vi "Results_filename_checker.vi"(4 "Filelength":i32=25, 5 "Warn if Already Exists":bool, 6 "Comment":string, 7 "Show Error handler":bool=TRUE, 8 "Results file":path) -> (0 "exists?":bool, 1 "Error String":string, 2 "cancelled":bool, 3 "Results file output":path)   [LabVIEW 2014]
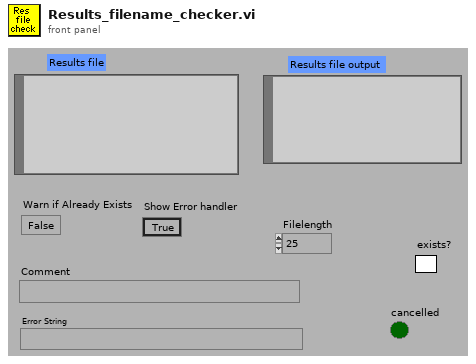
[diagram p1: front panel]
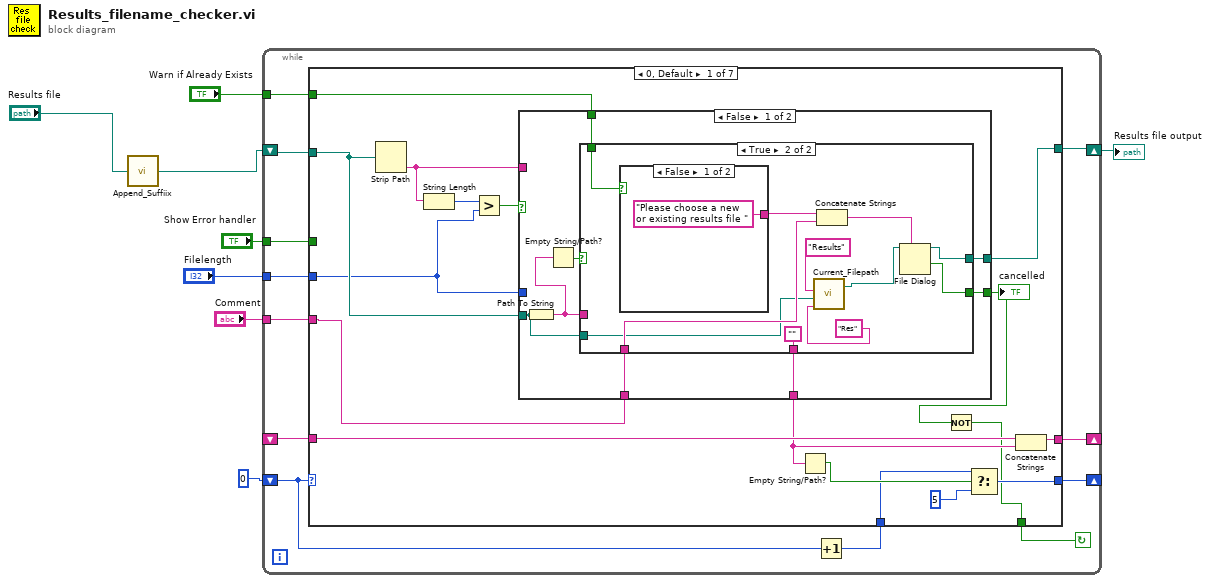
[diagram p0: block diagram]
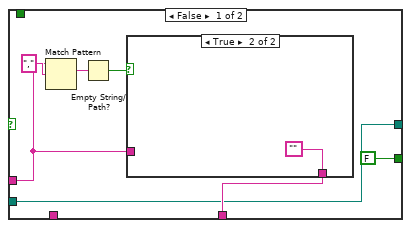
[diagram p2: hidden frame]
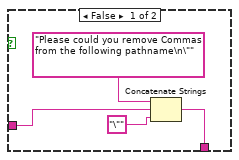
[diagram p3: hidden frame]
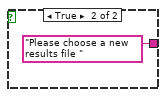
[diagram p4: hidden frame]
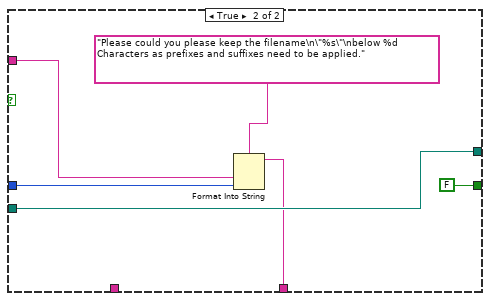
[diagram p5: hidden frame]
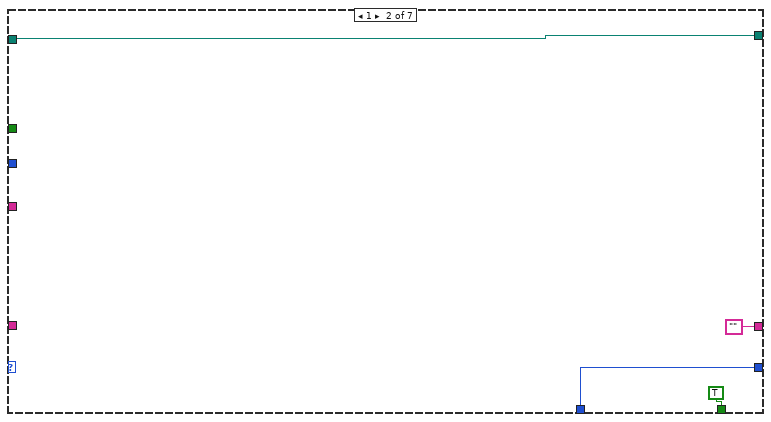
[diagram p6: hidden frame]
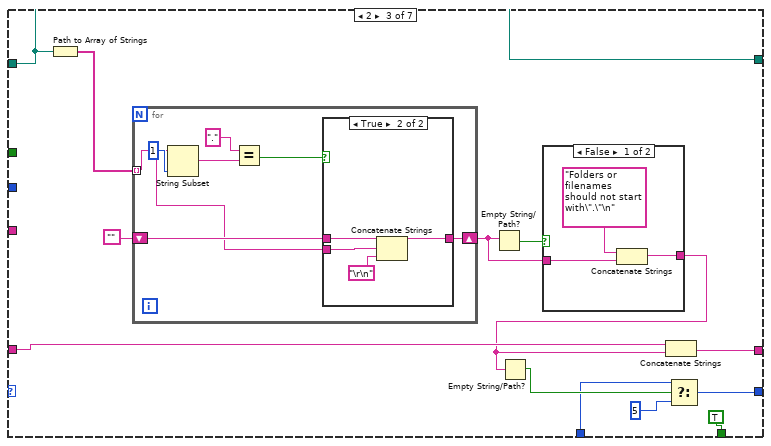
[diagram p7: hidden frame]
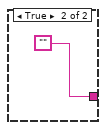
[diagram p8: hidden frame]
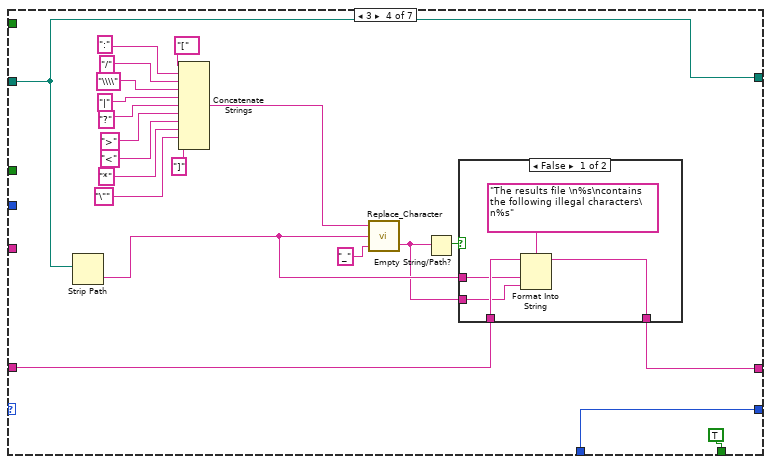
[diagram p10: hidden frame]
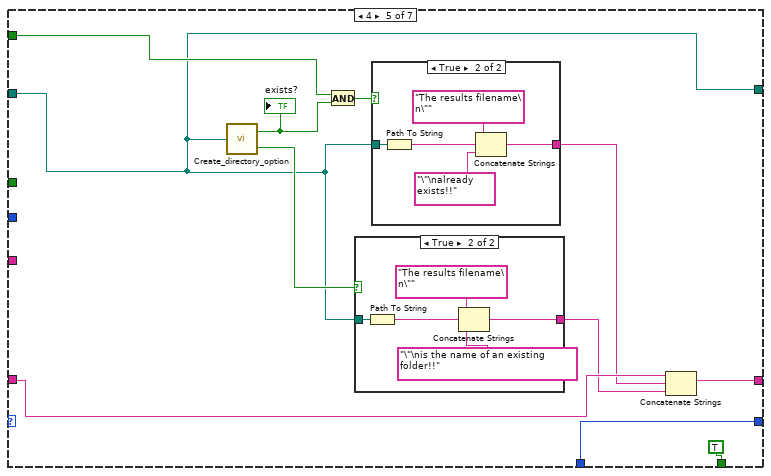
[diagram p12: hidden frame]
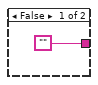
[diagram p13: hidden frame]
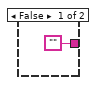
[diagram p14: hidden frame]
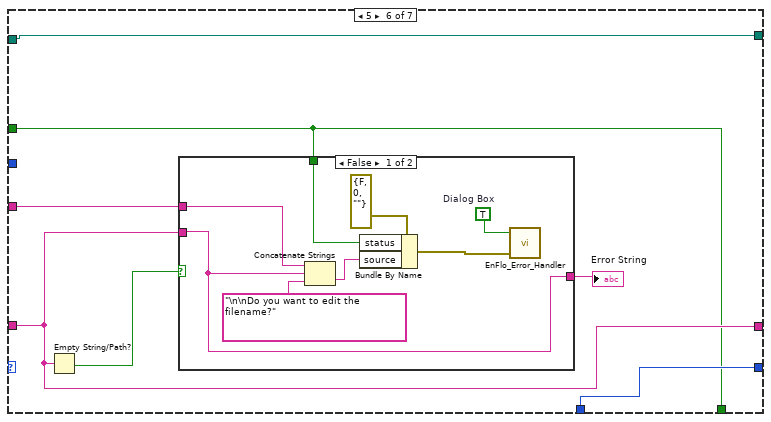
[diagram p15: hidden frame]
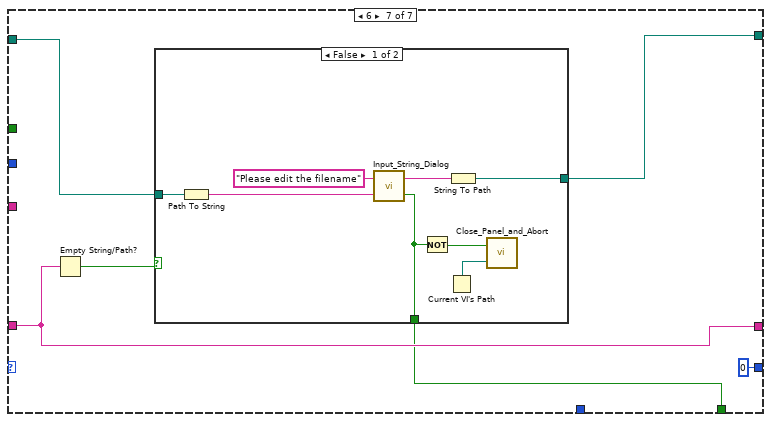
[diagram p17: hidden frame]
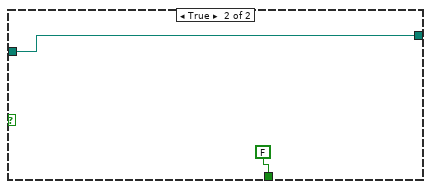
[diagram p18: hidden frame]
diagram:
  n1 = call "Append_Suffiix.vi"("Results file"="Results file") -> ("appended path"=w1:path)
  n2 = while {
    shift-left: 0 -> [w16]
    shift-right: [w12] -> _
    shift-left: _ -> [w15]
    shift-right: [w14] -> _
    tunnel: "Show Error handler" -> [w17]
    shift-left: w1 -> [w20]
    shift-right: [w19] -> w8
    tunnel: "Warn if Already Exists" -> [w11]
    tunnel: "Comment" -> [w10]
    tunnel: "Filelength" -> [w9]
    stop <- w18 continue-if-true
    n3 = Increment(x=w16) -> (x+1=w13:i32)
    n4 = case shown="0, Default" w16 {
      tunnel: w20 -> [w26 w77 w81 w117 w137 w161 w180]
      tunnel: [w27 w77 w81 w117 w137 w161 w181] -> w19
      tunnel: [w23 TRUE ("Ok Out") TRUE ("Ok Out") TRUE ("Ok Out") TRUE ("Ok Out") w162 w178] -> w18
      tunnel: w17 -> [_ _ _ _ _ w162 _]
      tunnel: w15 -> [w36 _ w86 w115 w144 w164 w179]
      tunnel: [w35 "" w84 w114 w143 w164 w179] -> w14
      tunnel: w13 -> [w32 w79 w83 w113 w141 w163 _]
      tunnel: [w30 w79 w82 w113 w141 w163 0 ("f")] -> w12
      tunnel: w11 -> [w25 _ _ _ w138 _ _]
      tunnel: w10 -> [w22 _ _ _ _ w160 _]
      tunnel: w9 -> [w21 _ _ _ _ _ _]
      frame 0, Default {
        n5 = Strip Path(path=w26) -> (name=w29:string)  [unwired: 1 out]
        n6 = String Length(string=w29) -> (length=w28:i32)
        n7 = Greater?(x=w28, y=w21) -> (0:w37:bool)
        n8 = case shown="False" w37 {
          tunnel: w26 -> [w41 w76]
          tunnel: w29 -> [_ w74]
          tunnel: [w45 w72] -> w34
          tunnel: [w42 w76] -> w27
          tunnel: w25 -> [w40 _]
          tunnel: [w39 FALSE ("cancelled")] -> w24
          tunnel: w22 -> [w38 _]
          tunnel: w21 -> [_ w73]
          frame False {
            n9 = Path To String(path=w41) -> (string=w44:string)
            n10 = Empty String/Path?(string/path=w44) -> (empty?=w43:bool)
            n11 = case shown="True" w43 {
              tunnel: [w52 ""] -> w45
              tunnel: w44 -> [w48 _]
              tunnel: [w47 w63] -> w42
              tunnel: w41 -> [w47 w60]
              tunnel: w40 -> [_ w67]
              tunnel: [FALSE ("cancelled") w62] -> w39
              tunnel: w38 -> [_ w65]
              frame False {
                n12 = Match Pattern(string=w48, regular expression=",") -> (match substring=w50:string)  [unwired: 4 out]
                n13 = Empty String/Path?(string/path=w50) -> (empty?=w49:bool)
                n14 = case shown="True" w49 {
                  tunnel: w48 -> [w55 _]
                  tunnel: [w54 ""] -> w52
                  frame False {
                    n15 = Concatenate Strings("Please could you remove Commas from the following pathname\n\"", w55, "\"") -> (w54:string)
                  }
                  frame True {
                  }
                }
              }
              frame True {
                n16 = case shown="False" w67 {
                  tunnel: ["Please choose a new or existing results file " ("prompt") "Please choose a new results file " ("prompt")] -> w66
                  frame False {
                  }
                  frame True {
                  }
                }
                n17 = call "Current_Filepath.vi"("Short_Name"="Res" ("Data Type"), "Filename in"=w60, "Data Type"="Results") -> ("Directory"=w59:path)  [unwired: 1 in, 1 out]
                n18 = Concatenate Strings(w66, w65) -> (w64:string)
                n19 = File Dialog(7:w64, 11:w59) -> (1:w62:bool, 3:w63:path)  [unwired: 5 in, 2 out]
              }
            }
          }
          frame True {
            n20 = Format Into String(format string="Please could you please keep the filename\n\"%s\"\nbelow %d Characters as prefixes and suffixes need to be applied.", w74, w73) -> (resulting string=w72:string)  [unwired: 2 in, 1 out]
          }
        }
        "cancelled" <- w24
        n21 = Empty String/Path?(string/path=w34) -> (empty?=w33:bool)
        n22 = Not(x=w24) -> (.not. x?=w23:bool)
        n23 = Select(t=w32, s=w33, f=5) -> (s? t:f=w30:i32)
        n24 = Concatenate Strings(w36, w34) -> (w35:string)
      }
      frame 1 {
      }
      frame 2 {
        n25 = Path to Array of Strings(0:w81) -> (2:w91:string[])  [unwired: 1 out]
        n26 = for {
          tunnel: w91 -> [w99] mode=indexing
          shift-right: [w98] -> w89
          shift-left: "" -> [w100]
          n27 = String Subset(string=w99, length (rest)=1 ("length")) -> (substring=w103:string)  [unwired: 1 out]
          n28 = Equal?(x=".", y=w103) -> (x = y?=w101:bool)
          n29 = case shown="True" w101 {
            tunnel: w100 -> [w105 w109]
            tunnel: w99 -> [_ w108]
            tunnel: [w105 w107] -> w98
            frame False {
            }
            frame True {
              n30 = Concatenate Strings(w109, w108, "\r\n") -> (w107:string)
            }
          }
        }
        n31 = Empty String/Path?(string/path=w89) -> (empty?=w90:bool)
        n32 = case shown="False" w90 {
          tunnel: [w94 ""] -> w85
          tunnel: w89 -> [w95 _]
          frame False {
            n33 = Concatenate Strings("Folders or filenames should not start with\".\"\n", w95) -> (w94:string)
          }
          frame True {
          }
        }
        n34 = Empty String/Path?(string/path=w85) -> (empty?=w88:bool)
        n35 = Concatenate Strings(w86, w85) -> (w84:string)
        n36 = Select(t=w83, s=w88, f=5) -> (s? t:f=w82:i32)
      }
      frame 3 {
        n37 = Strip Path(path=w117) -> (name=w111:string)  [unwired: 1 out]
        n38 = Concatenate Strings("[" ("Substring"), ":", "/", "\\\\", "|", "?", ">", "<", "*", "\"", "]" ("Substring")) -> (w119:string)
        n39 = call "Replace_Character.vi"("Replace with"="_", "Input String"=w111, "Search For"=w119) -> ("Matched Characters"=w110:string)  [unwired: 1 out]
        n40 = Empty String/Path?(string/path=w110) -> (empty?=w116:bool)
        n41 = case shown="False" w116 {
          tunnel: w115 -> [w134 w136]
          tunnel: [w133 w136] -> w114
          tunnel: w111 -> [w132 _]
          tunnel: w110 -> [w131 _]
          frame False {
            n42 = Format Into String(format string="The results file \n%s\ncontains the following illegal characters\n%s" ("Format String"), initial string=w134, w132, w131) -> (resulting string=w133:string)  [unwired: 1 in, 1 out]
          }
          frame True {
          }
        }
      }
      frame 4 {
        n43 = call "Create_directory_option.vi"("Filename"=w137) -> ("Path is to existing File"=w146:bool, "Path is to existing Directory"=w139:bool)
        "exists?" <- w146
        n44 = And(x=w138, y=w146) -> (x .and. y?=w145:bool)
        n45 = case shown="True" w139 {
          tunnel: w137 -> [_ w151]
          tunnel: ["" w150] -> w140
          frame False {
          }
          frame True {
            n46 = Path To String(path=w151) -> (string=w149:string)
            n47 = Concatenate Strings("The results filename\n\"", w149, "\"\nis the name of an existing folder!!") -> (w150:string)
          }
        }
        n48 = case shown="True" w145 {
          tunnel: w137 -> [_ w157]
          tunnel: ["" w156] -> w142
          frame False {
          }
          frame True {
            n49 = Path To String(path=w157) -> (string=w155:string)
            n50 = Concatenate Strings("The results filename\n\"", w155, "\"\nalready exists!!") -> (w156:string)
          }
        }
        n51 = Concatenate Strings(w144, w142, w140) -> (w143:string)
      }
      frame 5 {
        n52 = Empty String/Path?(string/path=w164) -> (empty?=w166:bool)
        n53 = case shown="False" w166 {
          tunnel: w164 -> [w168 w175]
          tunnel: [w168 w175] -> w165
          tunnel: w162 -> [w170 _]
          tunnel: w160 -> [w167 _]
          frame False {
            w172 = TRUE  # Dialog Box
            n54 = Concatenate Strings(w167, w168, "\n\nDo you want to edit the filename?") -> (w169:string)
            n55 = Bundle By Name(cluster=errorcluster {"status"=FALSE, "code"=0, "source"=""} ("error in (no error)"), "status"=w170, "source"=w169) -> (w173:errorcluster)
            n56 = call "EnFlo_Error_Handler.vi"("error in (no error)"=w173, "Dialog Box (T)"=w172) -> ()  [unwired: 1 in, 3 out]
          }
          frame True {
          }
        }
        "Error String" <- w165
      }
      frame 6 {
        n57 = Empty String/Path?(string/path=w179) -> (empty?=w176:bool)
        n58 = case shown="False" w176 {
          tunnel: [w182 w190] -> w181
          tunnel: [w184 FALSE ("Ok Out")] -> w178
          tunnel: w180 -> [w187 w190]
          frame False {
            n59 = Path To String(path=w187) -> (string=w183:string)
            n60 = call "Input_String_Dialog.vi"("Value"=w183, "Message to user"="Please edit the filename") -> ("Ok Out"=w184:bool, "Output string"=w188:string)
            n61 = Not(x=w184) -> (.not. x?=w186:bool)
            n62 = Current VI's Path() -> (path=w185:path)
            n63 = String To Path(string=w188) -> (path=w182:path)
            n64 = call "Close_Panel_and_Abort.vi"("Vi path"=w185, "stop"=w186) -> ()  [unwired: 1 out]
          }
          frame True {
          }
        }
      }
    }
  }
  "Results file output" <- w8
